vi "FinalProject.vi"() -> ()   [LabVIEW 2020]
uses:
  Keypad.ctl
  <vilib>/userdefined/High Color/IMAQdx.ctl
  Security_States.ctl
  <vilib>/MakerHub/LINX/Public/Utilities/Open Serial.vi
  <vilib>/MakerHub/LINX/Public/Sensors/Motion/Servo/Servo Open One Channel.vi
  <vilib>/MakerHub/LINX/Public/Sensors/Motion/Servo/Servo Close One Channel.vi
  <vilib>/MakerHub/LINX/LMH-LINX.lvlib
  <vilib>/MakerHub/LINX/Public/Sensors/Motion/Servo/Servo.lvlib
  <vilib>/vision/driver/NI_Vision_Acquisition_Software.lvlib
panel:
  in  "Boolean":bool caption="Up - Armed\nDown - Unarmed"
  out "New Password":string
  in  "Change Password":bool
  out "Password":string="12345"
  out "Response":u8[](array[numeric])
  in  "RFID":bool
  out "Image":T1(plugin-control)
  in  "Session In":T2
  in  "QR":bool
  in  "Serial Port":refnum<visa-resource-name>="N/A"
  in  "Password":string
  in  "Email":string
  in  "Phone Number":string
  in  "Carrier":enum16{"Sprint", "Verizon", "AT&T", "T-Mobile"}(ring)
  in  "Keypad":T3
  out "Door":u16[](array[ring])
  in  "stop":bool
  out "Alert":bool
  out "Red LED":bool
  out "Green LED":bool
  out "Password Display":string
  # "Set up text alert system"
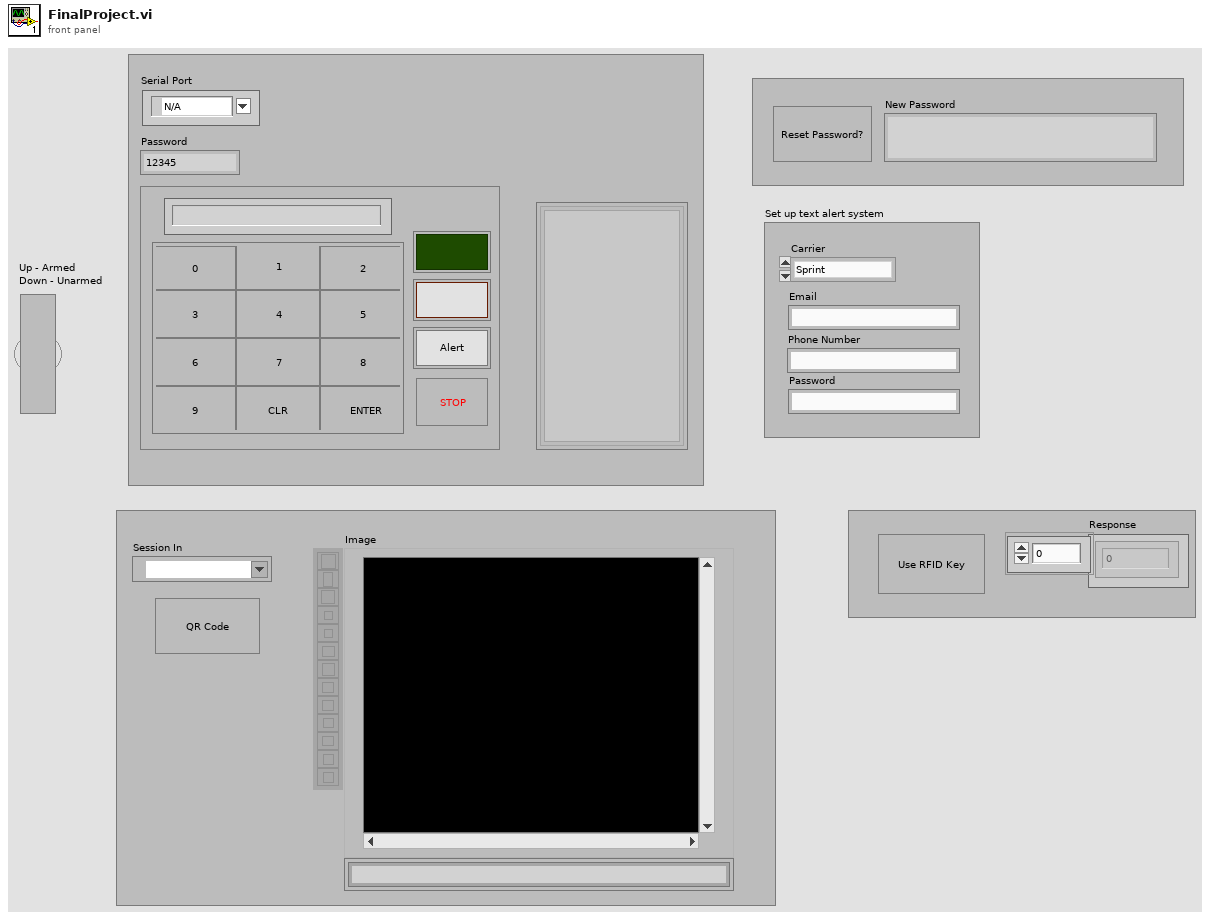
[diagram p1: front panel]
types:
  T1 = typedef "IMAQ Image.ctl" = refnum<image>
  T2 = typedef "IMAQdx.ctl" = refnum<k21>
  T3 = typedef "Keypad.ctl" = cluster{"0":bool, "1":bool, "2":bool, "3":bool, "4":bool, "5":bool, "6":bool, "7":bool, "8":bool, "9":bool, "CLR":bool, "Enter":bool}
  T4 = typedef "Security_States.ctl" = enum16{"Initialize", "Wait For Input", "Clear", "Check Password", "Correct", "Arming", "Password Reset ", "RFID", "QR Code", "Incorrect", "Alert"}
  T5 = typedef "LMH-LINX.lvlib/LINX Ref.ctl" = cluster{"IO":T6, "Interface":T7, "LINX Device Config":T8}
  T6 = typedef "LMH-LINX.lvlib/Platform.ctl" = enum16{"Remote", "Local"}
  T7 = typedef "LMH-LINX.lvlib/Interface.ctl" = enum16{"Serial", "TCP"}
  T8 = typedef "LMH-LINX.lvlib/Device.lvlib/LINX Device Config.ctl" = cluster{"Interface":T7, "COM Port":refnum<visa-resource-name>, "TCP Configuration":T9, "Device Family":u8, "Device ID":u8, "Device Name":string, "TCP Ref":refnum<k5>, "Channels":T10}
  T9 = typedef "LMH-LINX.lvlib/Device.lvlib/TCP Config.ctl" = cluster{"IP Address":string, "Port":u16}
  T10 = typedef "LMH-LINX.lvlib/Channels.ctl" = cluster{"DI":u8[], "DO":u8[], "AI":u8[], "AO":u8[], "PWM":u8[], "QE":u8[], "UART":u8[], "I2C 2":u8[], "SPI":u8[], "CAN":u8[], "Servo":u8[], "AI Ref (V)":dbl, "AI Resolution (Bits)":u8, "AO Ref (V)":dbl, "AO Resolution (Bits)":u8}
  T11 = enum8{"Enabled", "Disabled", "Disabled and Grayed Out"}
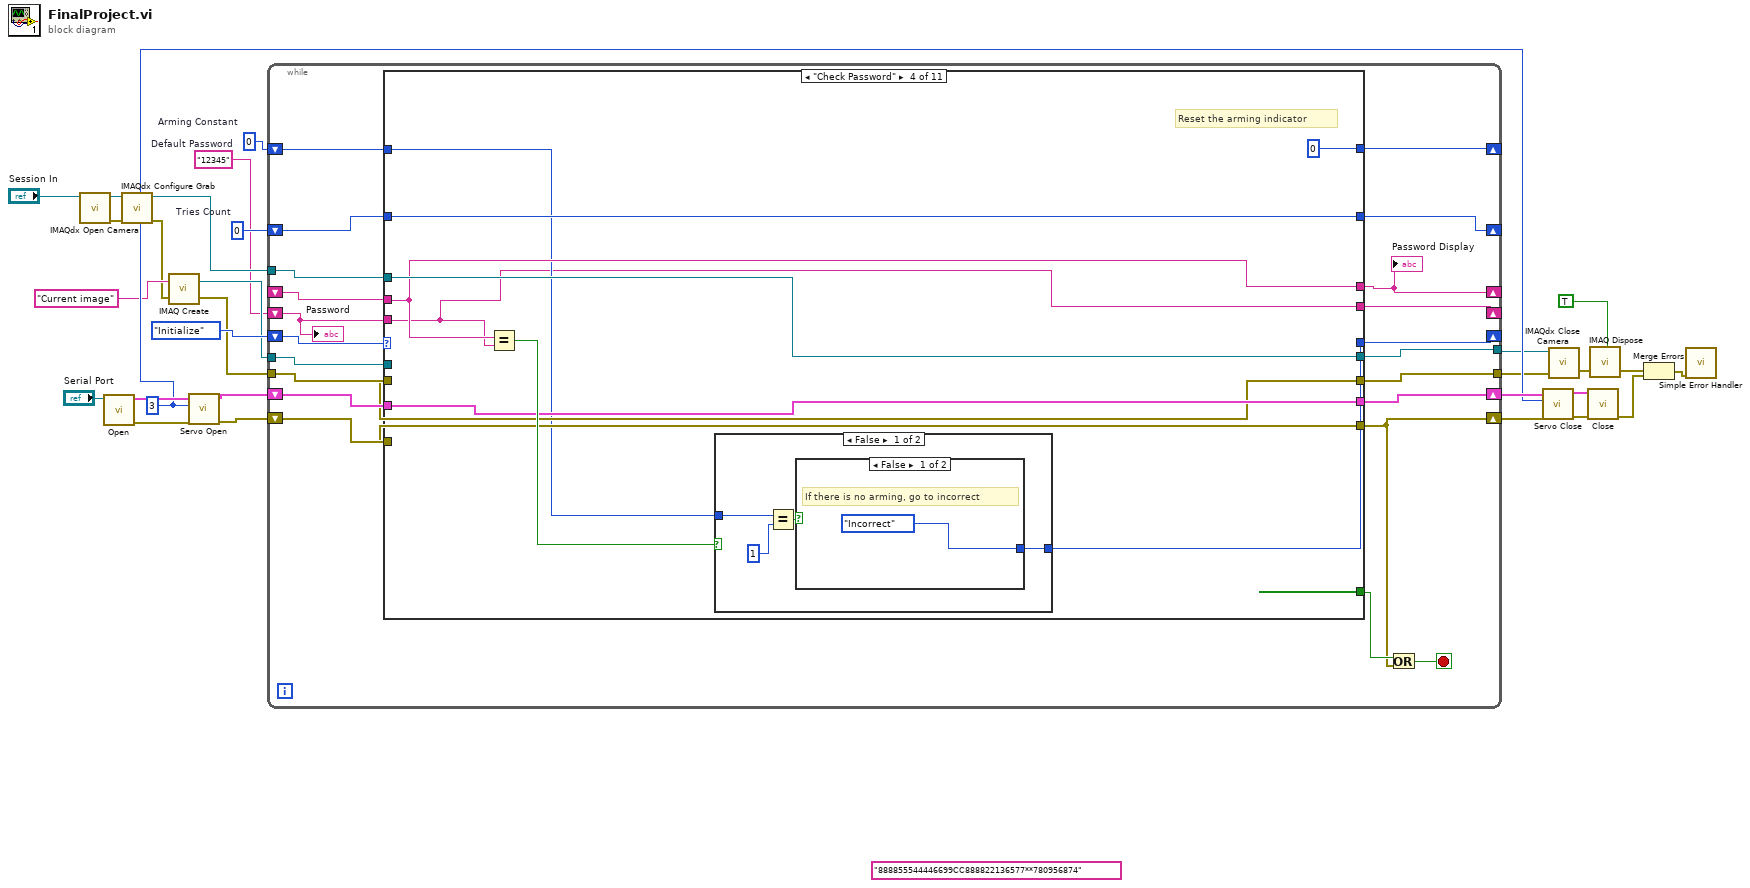
[diagram p0: block diagram]
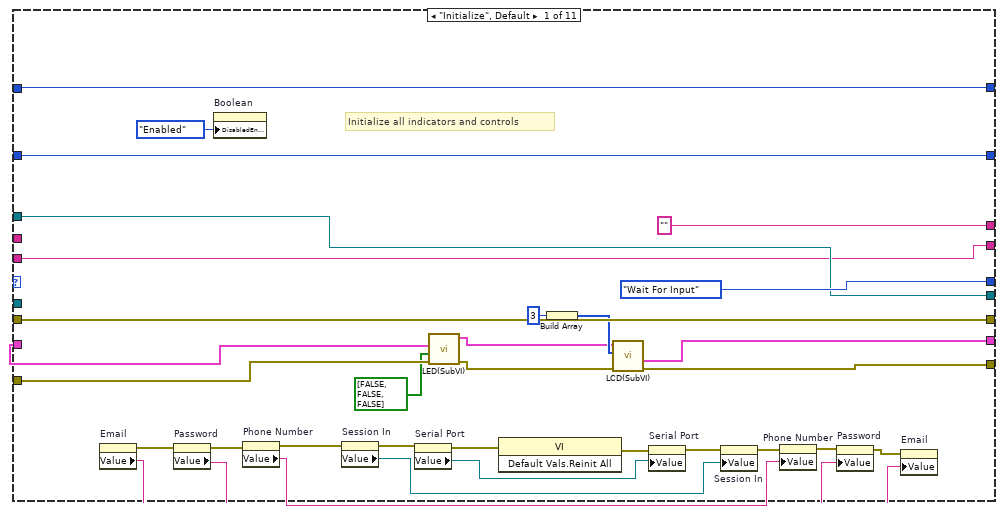
[diagram p2: hidden frame]
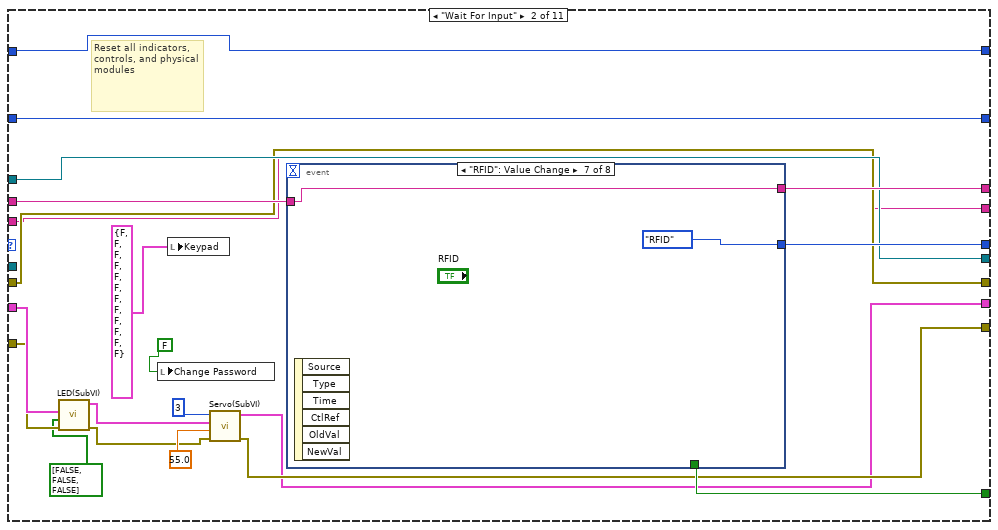
[diagram p3: hidden frame]
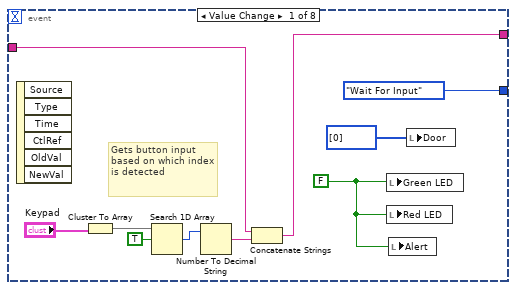
[diagram p4: hidden frame]
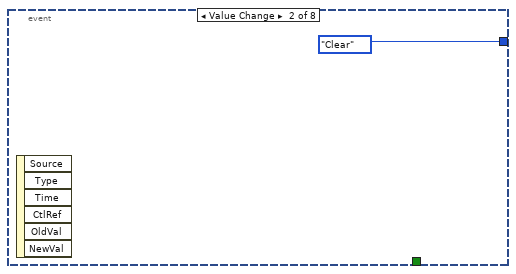
[diagram p5: hidden frame]
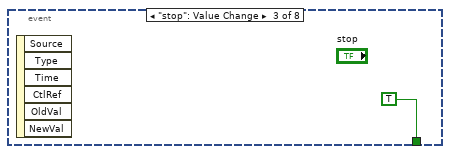
[diagram p6: hidden frame]
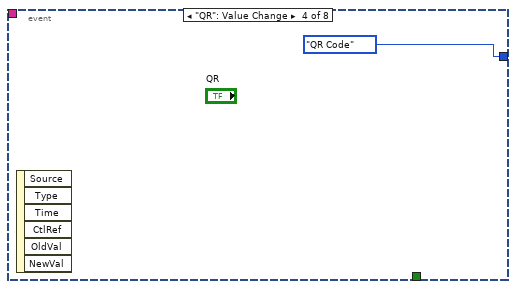
[diagram p7: hidden frame]
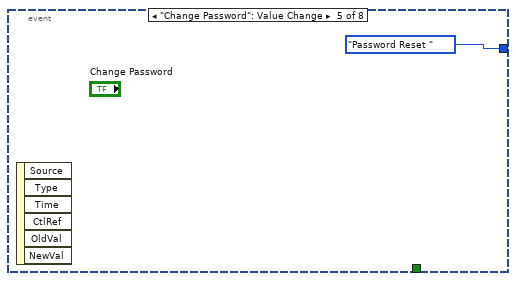
[diagram p8: hidden frame]
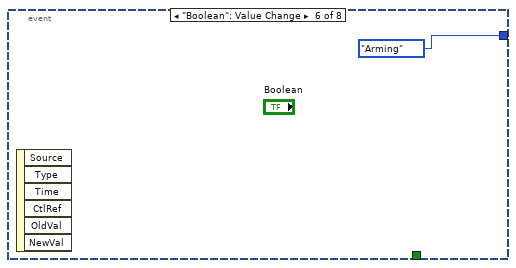
[diagram p9: hidden frame]
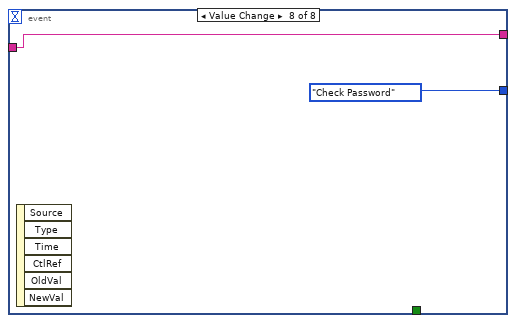
[diagram p10: hidden frame]
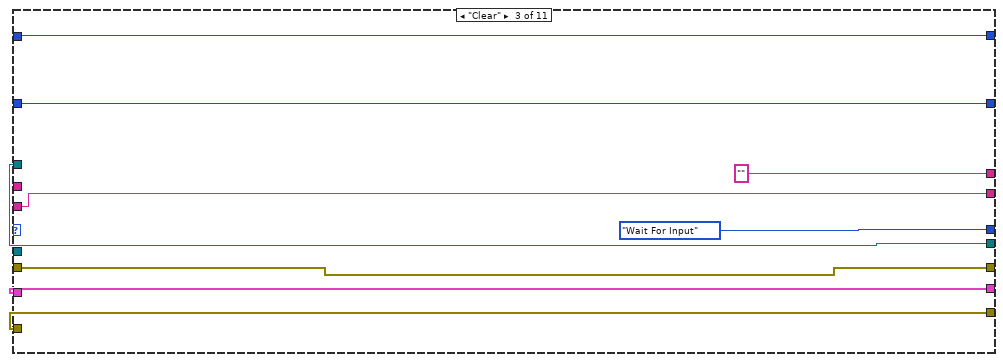
[diagram p11: hidden frame]
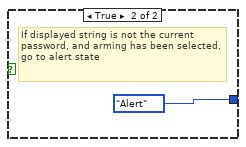
[diagram p12: hidden frame]
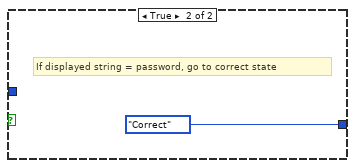
[diagram p13: hidden frame]
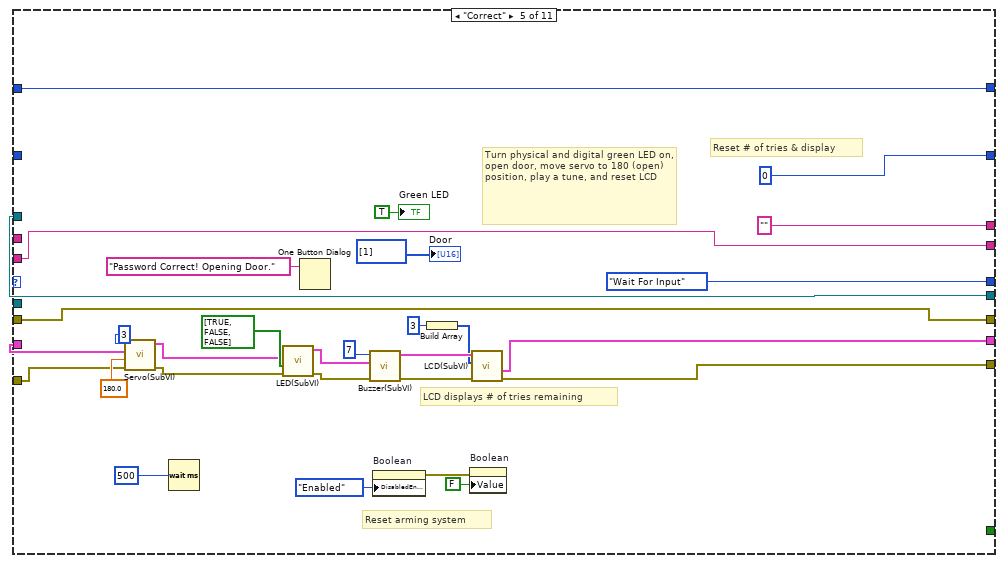
[diagram p14: hidden frame]
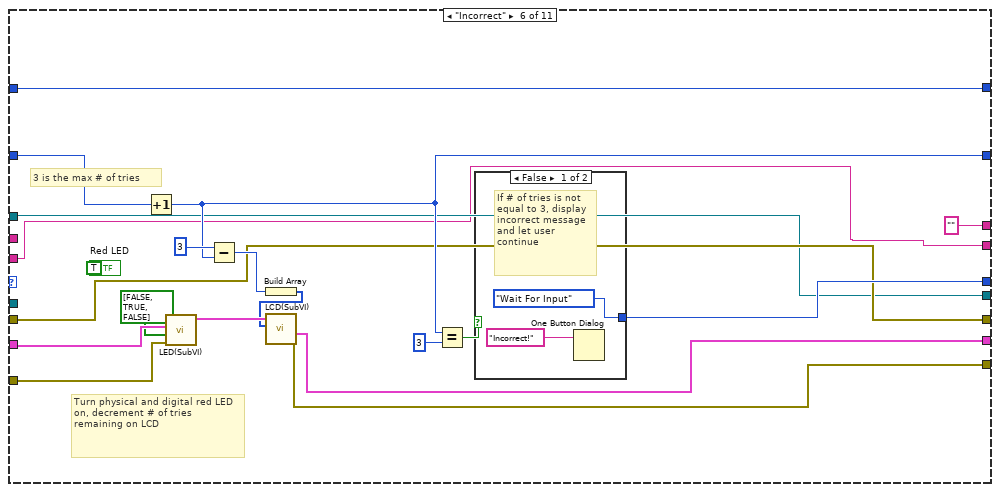
[diagram p15: hidden frame]
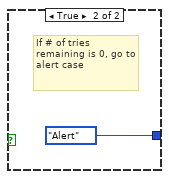
[diagram p16: hidden frame]
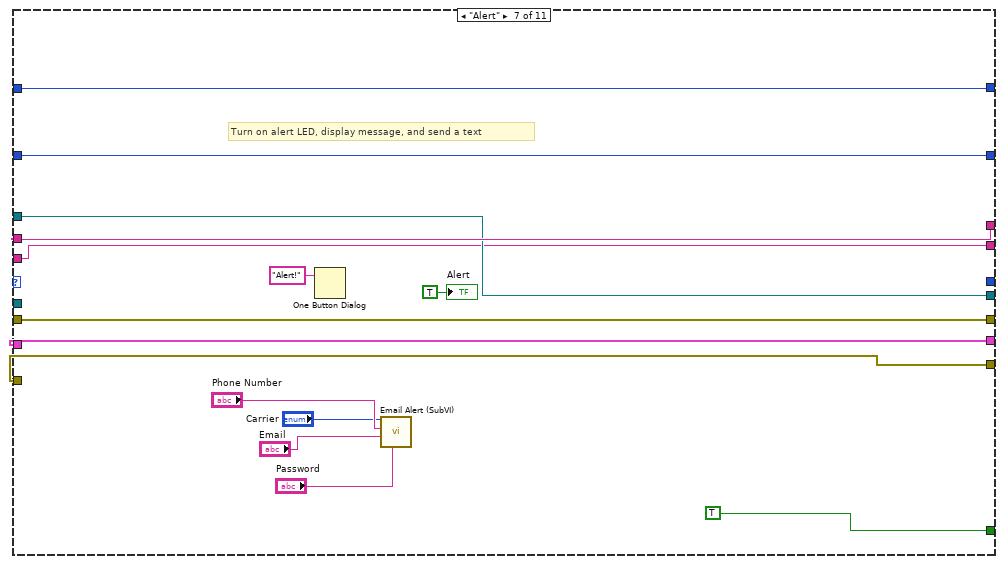
[diagram p17: hidden frame]
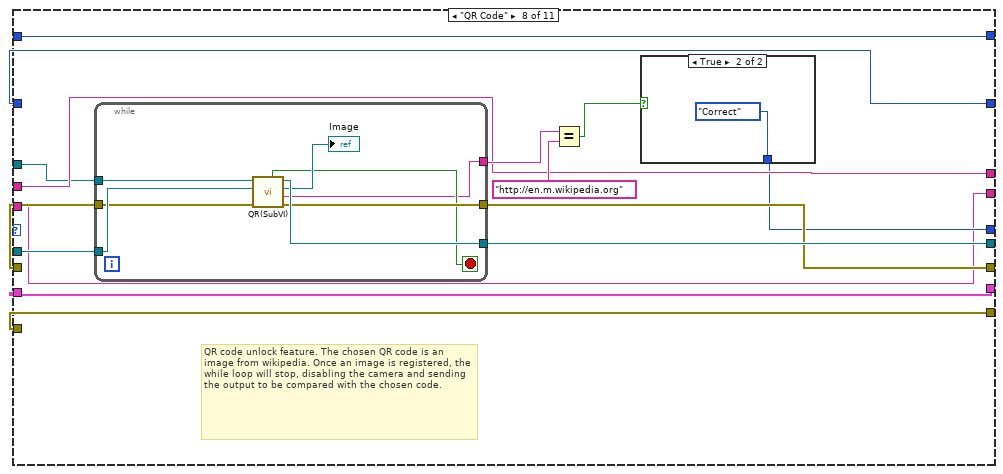
[diagram p18: hidden frame]
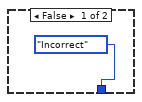
[diagram p19: hidden frame]
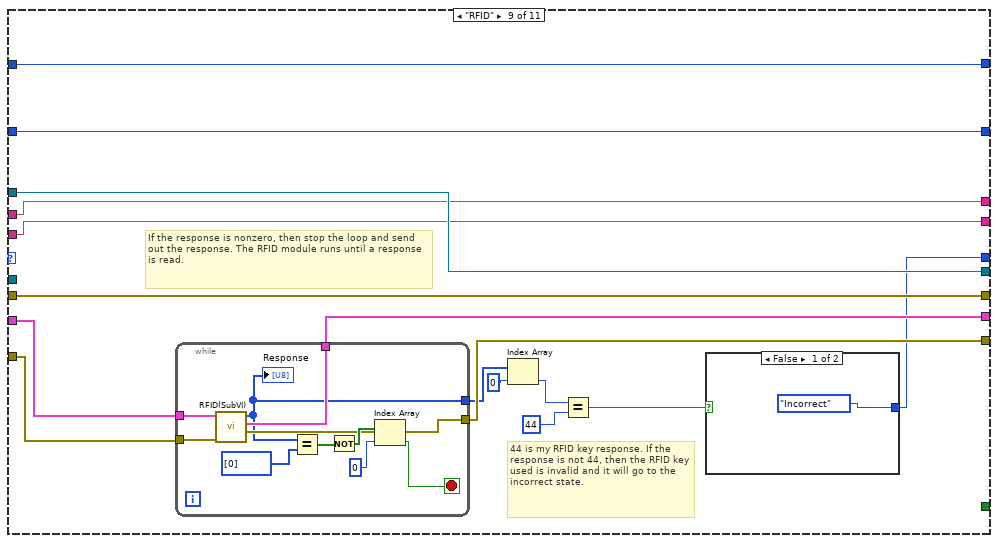
[diagram p20: hidden frame]
diagram:
  w1 = 0  # Arming Constant
  (unwired) "888855544446699CC888822136577**780956874" ("string")
  w2 = "12345"  # Default Password
  w18 = u8 3 ("Servo Channel")
  w28 = u8 0  # Tries Count
  n1 = call <vilib>:"IMAQdx Open Camera.vi"("Session In"="Session In") -> ("error out"=w15:errorcluster, "Session Out"=w16:T2)  [unwired: 9 in]
  n2 = call-poly <vilib>:"Open.vi"("Serial Port"="Serial Port") -> ("Error Out"=w24:errorcluster, "LINX Resource"=w26:T5)  [unwired: 8 in, 1 out]
  n3 = call <vilib>:"IMAQdx Configure Grab.vi"("error in"=w15, "Session In"=w16) -> ("error out"=w13:errorcluster, "Session Out"=w12:T2)  [unwired: 8 in]
  n4 = call "IMAQ Create"("Image Name"="Current image", "error in (no error)"=w13) -> ("New Image"=w11:T1, "error out"=w10:errorcluster)  [unwired: 3 in]
  n5 = call-poly <vilib>:"Servo Open.vi"("Error In"=w24, "Servo Channel"=w18, "LINX Resource"=w26) -> ("Error Out"=w23:errorcluster, "LINX Resource"=w25:T5)  [unwired: 7 in]
  n6 = while {
    shift-right: [w48] -> _
    shift-left: Security_States."Initialize" -> [w50]
    shift-right: [w34] -> _
    shift-left: _ -> [w49]
    shift-right: [w46] -> _
    shift-left: w28 -> [w47]
    shift-right: [w43] -> w22
    shift-left: w25 -> [w45]
    shift-right: [w40] -> w21
    shift-left: w23 -> [w44]
    tunnel: w12 -> [w39]
    tunnel: w11 -> [w35]
    tunnel: w10 -> [w38]
    tunnel: [w37] -> w7
    tunnel: [w36] -> w6
    shift-right: [w32] -> _
    shift-left: w2 -> [w33]
    shift-right: [w30] -> _
    shift-left: w1 -> [w31]
    stop <- w42 stop-if-true
    n7 = case shown="\"Check Password\"" w50 {
      tunnel: ["" ("Number Display") w102 "" ("Number Display") w134 "" ("Number Display") "" ("Number Display") w214 w222 w244 w281 w321] -> w34
      tunnel: w49 -> [_ w94 _ w134 _ _ w214 w222 w244 w281 w321]
      tunnel: [Security_States."Wait For Input" w101 Security_States."Wait For Input" w140 Security_States."Wait For Input" w196 _ w220 w245 Security_States."Wait For Input" Security_States."Wait For Input"] -> w48
      tunnel: w47 -> [w80 w100 w128 w139 _ w186 w204 w223 w257 w282 w320]
      tunnel: [w80 w100 w128 w139 u8 0 w183 w204 w223 w257 w282 w320] -> w46
      tunnel: [_ w99 _ _ _ _ TRUE ("x") _ _ _ _] -> w41
      tunnel: w45 -> [w79 w98 w127 w138 w162 w193 w208 w231 w254 w278 w319]
      tunnel: w44 -> [w78 w97 w126 w137 w154 w192 w207 w230 w253 w277 w318]
      tunnel: [w67 w88 w127 w138 w159 w189 w208 w231 w252 w276 w319] -> w43
      tunnel: [w66 w89 w126 w137 w158 w188 w207 w230 w251 w275 w318] -> w40
      tunnel: w39 -> [w72 w95 w124 w135 w155 w181 w205 w219 w256 w280 w317]
      tunnel: w38 -> [w73 w87 w125 w136 w156 w182 w206 w228 w255 w279 w316]
      tunnel: [w72 w95 w124 w135 w155 w181 w205 w227 w256 w280 w317] -> w37
      tunnel: [w73 w87 w125 w136 w156 w182 w206 w226 w255 w279 w316] -> w36
      tunnel: w35 -> [_ _ _ _ _ _ _ w229 _ _ _]
      tunnel: w33 -> [w62 w86 w123 w131 w153 w180 w203 w218 w243 _ w315]
      tunnel: [w62 w86 w123 w131 w153 w180 w203 w218 w243 w274 w315] -> w32
      tunnel: w31 -> [w61 w83 w122 w133 w152 w179 w202 w217 w242 w270 w313]
      tunnel: [w61 w83 w122 0 w152 w179 w202 w217 w242 w270 w312] -> w30
      frame "Initialize", Default {
        # "Initialize all indicators and controls"
        n8 = property on="Email" class="Str"() -> (error out=w52:errorcluster, "Value"=w51:string)  [unwired: 2 in, 1 out]
        n9 = property on="Password" class="Str"(error in=w52) -> (error out=w56:errorcluster, "Value"=w54:string)  [unwired: 1 in, 1 out]
        n10 = property on="Boolean" class="Bool (strict)"("DisabledEnum"=T11."Enabled" ("Disabled")) -> ()  [unwired: 2 in, 2 out]
        n11 = property on="Phone Number" class="Str"(error in=w56) -> (error out=w59:errorcluster, "Value"=w58:string)  [unwired: 1 in, 1 out]
        n12 = property on="Session In" class="IMAQdx (strict)"(error in=w59) -> (error out=w65:errorcluster, "Value"=w63:T2)  [unwired: 1 in, 1 out]
        n13 = property on="Serial Port" class="VISAName"(error in=w65) -> (error out=w76:errorcluster, "Value"=w74:refnum<visa-resource-name>)  [unwired: 1 in, 1 out]
        n14 = call "LED(SubVI).vi"("error in (no error)"=w78, "Values"=bool[] [FALSE, FALSE, FALSE], "LINX Resource in"=w79) -> ("error out"=w68:errorcluster, "LINX Resource out"=w69:T5)  [unwired: 7 in]
        n15 = invoke class="VI" method="Default Vals.Reinit All"(error in=w76) -> (error out=w75:errorcluster)  [unwired: 2 in, 2 out]
        n16 = Build Array(u8 3 ("element")) -> (w70:u8[])
        n17 = call "LCD(SubVI).vi"("error in (no error)"=w68, "Data"=w70, "LINX Resource in"=w69) -> ("error out"=w66:errorcluster, "LINX Resource out"=w67:T5)  [unwired: 4 in, 3 out]
        n18 = property on="Serial Port" class="VISAName"(error in=w75, "Value"=w74) -> (error out=w64:errorcluster)  [unwired: 1 in, 1 out]
        n19 = property on="Session In" class="IMAQdx (strict)"(error in=w64, "Value"=w63) -> (error out=w57:errorcluster)  [unwired: 1 in, 1 out]
        n20 = property on="Phone Number" class="Str"(error in=w57, "Value"=w58) -> (error out=w55:errorcluster)  [unwired: 1 in, 1 out]
        n21 = property on="Password" class="Str"(error in=w55, "Value"=w54) -> (error out=w53:errorcluster)  [unwired: 1 in, 1 out]
        n22 = property on="Email" class="Str"(error in=w53, "Value"=w51) -> ()  [unwired: 1 in, 2 out]
      }
      frame "Wait For Input" {
        # "Reset all indicators, controls, and physical modules"
        n23 = call "LED(SubVI).vi"("error in (no error)"=w97, "Values"=bool[] [FALSE, FALSE, FALSE], "LINX Resource in"=w98) -> ("error out"=w90:errorcluster, "LINX Resource out"=w91:T5)  [unwired: 7 in]
        n24 = local write "Change Password"(FALSE ("Enter")) -> ()
        n25 = local write "Keypad"(T3 {"0"=FALSE, "1"=FALSE, "2"=FALSE, "3"=FALSE, "4"=FALSE, "5"=FALSE, "6"=FALSE, "7"=FALSE, "8"=FALSE, "9"=FALSE, "CLR"=FALSE, "Enter"=FALSE} ("Keypad")) -> ()
        n26 = call "Servo(SubVI).vi"("error in (no error)"=w90, "Position"=55.0, "LINX Resource in"=w91, "Servo Channel"=u8 3) -> ("error out"=w89:errorcluster, "LINX Resource out"=w88:T5)  [unwired: 6 in]
        n27 = event shown="[6] \"RFID\": Value Change" {
          selector: _ -> [_ _ _ _ _ _ _ _]
          dyn-events: _ -> [_ _ _ _ _ _ _ _]
          timeout: _ -> [_ _ _ _ _ _ _ _]
          tunnel: [w109 _ _ _ _ _ w118 w120] -> w102
          tunnel: [Security_States."Wait For Input" Security_States."Clear" _ Security_States."QR Code" Security_States."Password Reset " Security_States."Arming" Security_States."RFID" Security_States."Check Password"] -> w101
          tunnel: [_ _ TRUE ("x") _ _ _ _ _] -> w99
          tunnel: w94 -> [w103 _ _ _ _ _ w118 w120]
          event Value Change {
            w104 = FALSE ("Green LED")
            # "Gets button input based on which index is detected"
            n28 = event-data() -> ()  [unwired: 1 in, 6 out]
            n29 = Cluster To Array(cluster="Keypad") -> (array=w107:bool[])
            n30 = Search 1D Array(1D array=w107, element=TRUE) -> (index of element=w111:i32)  [unwired: 1 in]
            n31 = Number To Decimal String(number=w111) -> (decimal integer string=w110:string)  [unwired: 1 in]
            n32 = Concatenate Strings(w103, w110) -> (w109:string)
            n33 = local write "Green LED"(w104) -> ()
            n34 = local write "Red LED"(w104) -> ()
            n35 = local write "Alert"(w104) -> ()
            n36 = local write "Door"(u16[] [0] ("Door")) -> ()
          }
          event Value Change {
            n37 = event-data() -> ()  [unwired: 1 in, 6 out]
          }
          event "stop": Value Change {
            n38 = event-data() -> ()  [unwired: 1 in, 6 out]
          }
          event "QR": Value Change {
            n39 = event-data() -> ()  [unwired: 1 in, 6 out]
          }
          event "Change Password": Value Change {
            n40 = event-data() -> ()  [unwired: 1 in, 6 out]
          }
          event "Boolean": Value Change {
            n41 = event-data() -> ()  [unwired: 1 in, 6 out]
          }
          event "RFID": Value Change {
            n42 = event-data() -> ()  [unwired: 1 in, 6 out]
          }
          event Value Change {
            n43 = event-data() -> ()  [unwired: 1 in, 6 out]
          }
        }
      }
      frame "Clear" {
      }
      frame "Check Password" {
        # "Reset the arming indicator"
        n44 = Equal?(x=w134, y=w131) -> (x = y?=w141:bool)
        n45 = case shown="False" w141 {
          tunnel: [w145 Security_States."Correct"] -> w140
          tunnel: w133 -> [w143 _]
          frame False {
            n46 = Equal?(x=w143, y=1) -> (x = y?=w144:bool)
            n47 = case shown="False" w144 {
              tunnel: [Security_States."Incorrect" Security_States."Alert"] -> w145
              frame False {
                # "If there is no arming, go to incorrect"
              }
              frame True {
                # "If displayed string is not the current password, and arming has been selected, go to alert state"
              }
            }
          }
          frame True {
            # "If displayed string = password, go to correct state"
          }
        }
      }
      frame "Correct" {
        # "Reset # of tries & display"
        # "Reset arming system"
        # "LCD displays # of tries remaining"
        # "Turn physical and digital green LED on, open door, move servo to 180 (open) position, play a tune, and reset LCD"
        n48 = call "Servo(SubVI).vi"("error in (no error)"=w154, "Position"=180.0, "LINX Resource in"=w162, "Servo Channel"=u8 3) -> ("error out"=w160:errorcluster, "LINX Resource out"=w161:T5)  [unwired: 6 in]
        n49 = Wait (ms)(milliseconds to wait=u32 500) -> ()  [unwired: 1 out]
        n50 = call "LED(SubVI).vi"("error in (no error)"=w160, "Values"=bool[] [TRUE, FALSE, FALSE], "LINX Resource in"=w161) -> ("error out"=w169:errorcluster, "LINX Resource out"=w170:T5)  [unwired: 7 in]
        n51 = One Button Dialog(message="Password Correct! Opening Door.") -> ()  [unwired: 1 in, 1 out]
        n52 = call "Buzzer(SubVI).vi"("error in (no error)"=w169, "LINX Resource in"=w170, "Buzzer Channel"=u8 7) -> ("error out"=w167:errorcluster, "LINX Resource out"=w168:T5)  [unwired: 7 in]
        n53 = property on="Boolean" class="Bool (strict)"("DisabledEnum"=T11."Enabled" ("Disabled")) -> (error out=w150:errorcluster)  [unwired: 2 in, 1 out]
        n54 = Build Array(u8 3 ("element")) -> (w165:u8[])
        n55 = property on="Boolean" class="Bool (strict)"(error in=w150, "Value"=FALSE ("Boolean")) -> ()  [unwired: 1 in, 2 out]
        n56 = call "LCD(SubVI).vi"("error in (no error)"=w167, "Data"=w165, "LINX Resource in"=w168) -> ("error out"=w158:errorcluster, "LINX Resource out"=w159:T5)  [unwired: 4 in, 3 out]
        "Green LED" <- TRUE ("Green LED")
        "Door" <- u16[] [1] ("Door")
      }
      frame "Incorrect" {
        # "Turn physical and digital red LED on, decrement # of tries remaining on LCD"
        # "3 is the max # of tries"
        n57 = Increment(x=w186) -> (x+1=w183:u8)
        n58 = call "LED(SubVI).vi"("error in (no error)"=w192, "Values"=bool[] [FALSE, TRUE, FALSE], "LINX Resource in"=w193) -> ("LINX Resource out"=w190:T5)  [unwired: 7 in, 1 out]
        n59 = Subtract(x=u8 3, y=w183) -> (x-y=w187:u8)
        n60 = Build Array(w187) -> (w184:u8[])
        n61 = call "LCD(SubVI).vi"("Data"=w184, "LINX Resource in"=w190) -> ("error out"=w188:errorcluster, "LINX Resource out"=w189:T5)  [unwired: 5 in, 3 out]
        n62 = Equal?(x=w183, y=u8 3) -> (x = y?=w197:bool)
        n63 = case shown="False" w197 {
          tunnel: [Security_States."Wait For Input" Security_States."Alert"] -> w196
          frame False {
            # "If # of tries is not equal to 3, display incorrect message and let user continue"
            n64 = One Button Dialog(message="Incorrect!") -> ()  [unwired: 1 in, 1 out]
          }
          frame True {
            # "If # of tries remaining is 0, go to alert case"
          }
        }
        "Red LED" <- TRUE ("Red LED")
      }
      frame "Alert" {
        # "Turn on alert LED, display message, and send a text"
        n65 = One Button Dialog(message="Alert!") -> ()  [unwired: 1 in, 1 out]
        n66 = call "Email Alert (SubVI).vi"("Password"="Password", "Email"="Email", "Phone Number"="Phone Number", "Carrier"="Carrier") -> ()  [unwired: 7 in, 1 out]
        "Alert" <- TRUE ("Alert")
      }
      frame "QR Code" {
        # "QR code unlock feature. The chosen QR code is an image from wikipedia. Once an image is registered, the while loop will stop, disabling the camera and sending the output to be compared with the chosen code."
        n67 = while {
          tunnel: w219 -> [w241]
          tunnel: w229 -> [w240]
          tunnel: w228 -> [w239]
          tunnel: [w238] -> w227
          tunnel: [w236] -> w226
          tunnel: [w234] -> w225
          stop <- w235 stop-if-true
          n68 = call "QR(SubVI).vi"("error in (no error)"=w239, "New Image"=w240, "Refnum in"=w241) -> ("error out"=w236:errorcluster, "Data"=w234:string, "Image"=→"Image":T1, "Refnum out"=w238:T2, "Found?"=w235:bool)  [unwired: 4 in]
        }
        n69 = Equal?(x=w225, y="http://en.m.wikipedia.org") -> (x = y?=w221:bool)
        n70 = case shown="True" w221 {
          tunnel: [Security_States."Incorrect" Security_States."Correct"] -> w220
          frame False {
          }
          frame True {
          }
        }
      }
      frame "RFID" {
        # "If the response is nonzero, then stop the loop and send out the response. The RFID module runs until a response is read."
        # "44 is my RFID key response. If the response is not 44, then the RFID key used is invalid and it will go to the incorrect state."
        n71 = while {
          tunnel: w254 -> [w269]
          tunnel: w253 -> [w268]
          tunnel: [w262] -> w252
          tunnel: [w261] -> w251
          tunnel: [w260] -> w249
          stop <- w263 stop-if-true
          n72 = call "RFID(SubVI).vi"("error in (no error)"=w268, "LINX Resource in"=w269) -> ("error out"=w261:errorcluster, "LINX Resource out"=w262:T5, "Response"=w260:u8[])  [unwired: 7 in]
          "Response" <- w260
          n73 = Equal?(x=w260, y=u8[] [0]) -> (x = y?=w266:bool[])
          n74 = Not(x=w266) -> (.not. x?=w265:bool[])
          n75 = Index Array(array=w265, index=0) -> (element=w263:bool)
        }
        n76 = Index Array(array=w249, index=0) -> (element=w247:u8)
        n77 = Equal?(x=w247, y=u8 44) -> (x = y?=w250:bool)
        n78 = case shown="False" w250 {
          tunnel: [Security_States."Incorrect" Security_States."Correct"] -> w245
          frame False {
          }
          frame True {
          }
        }
      }
      frame "Password Reset " {
        n79 = flat-sequence {
          tunnel: w278 -> [w289]
          tunnel: w277 -> [w288]
          tunnel: [w287] -> w273
          tunnel: [w286] -> w272
          tunnel: [w284] -> w271
          tunnel: [w308] -> w274
          tunnel: [w309] -> w275
          tunnel: [w310] -> w276
          tunnel: w273 -> [w310]
          tunnel: w272 -> [w309]
          tunnel: w271 -> [w308]
          frame #0 {
            n80 = while {
              shift-right: [w301] -> w286
              shift-left: w288 -> [w303]
              shift-right: [w302] -> w287
              shift-left: w289 -> [w304]
              shift-right: [w294] -> _
              shift-left: "" -> [w295]
              tunnel: [w294] -> w284
              stop <- w290 stop-if-true
              # "If new string != previous string + ÿ, print the new string. If they are the same, don't print anything"
              # "Stop when 5 numbers have been read"
              n81 = Concatenate Strings(w295, "ÿ" ("string")) -> (w298:string)
              n82 = call "4x4Keys(SubVI).vi"("error in (no error)"=w303, "LINX Resource in"=w304) -> ("error out"=w301:errorcluster, "LINX Resource out"=w302:T5, "string"=w296:string)  [unwired: 6 in, 1 out]
              n83 = Concatenate Strings(w295, w296) -> (w297:string)
              n84 = Equal?(x=w298, y=w297) -> (x = y?=w300:bool)
              n85 = case shown="False" w300 {
                tunnel: w297 -> [w305 _]
                tunnel: [w305 w306] -> w294
                tunnel: w295 -> [_ w306]
                frame False {
                  "New Password" <- w305
                }
                frame True {
                }
              }
              n86 = String To Byte Array(string=w294) -> (unsigned byte array=w293:u8[])
              n87 = Array Size(array=w293) -> (size(s)=w292:i32)
              n88 = Equal?(x=w292, y=5) -> (x = y?=w290:bool)
            }
          }
          frame #1 {
            n89 = One Button Dialog(message="Password has been reset!") -> ()  [unwired: 1 in, 1 out]
          }
        }
      }
      frame "Arming" {
        # "Increment arming constant to indicate that system has been armed"
        n90 = Increment(x=w313) -> (x+1=w312:i32)
        n91 = property on="Boolean" class="Bool (strict)"("DisabledEnum"=T11."Disabled and Grayed Out" ("Disabled")) -> ()  [unwired: 2 in, 2 out]
      }
    }
    "Password Display" <- w34
    n92 = Or(x=w41, y=w40) -> (x .or. y?=w42:bool)
    "Password" <- w33
  }
  n93 = call-poly <vilib>:"Servo Close.vi"("Error In"=w21, "Servo Channel"=w18, "LINX Resource"=w22) -> ("Error Out"=w19:errorcluster, "LINX Resource"=w20:T5)  [unwired: 7 in]
  n94 = call <vilib>:"IMAQdx Close Camera.vi"("error in"=w6, "Session In"=w7) -> ("error out"=w9:errorcluster)  [unwired: 9 in]
  n95 = call <vilib>:"Close.vi"("Error In"=w19, "LINX Resource"=w20) -> ("Error Out"=w4:errorcluster)  [unwired: 9 in]
  n96 = call "IMAQ Dispose"("All Images? (No)"=TRUE, "error in (no error)"=w9) -> ("error out"=w5:errorcluster)  [unwired: 4 in]
  n97 = Merge Errors(w5, w4) -> (w3:errorcluster)
  n98 = call <vilib>:"Simple Error Handler.vi"("error in (no error)"=w3) -> ()  [unwired: 4 in, 5 out]
